vi "Digital Write.vi"(8 "Error In":errorcluster, 9 "Values":bool[](array[boolean]), 10 "Channels":u8[](array[numeric]), 11 "LINX Device Config":T1) -> (0 "Error Out":errorcluster, 3 "LINX Device Config":T1)   [LabVIEW 2013, in "LVH-LINX.lvlib" / "Device.lvlib"]
doc: "Set the value of one or more digital output pin."
uses:
  <vilib>/LabVIEW Hacker/LINX/Private/Device/Device.lvlib
  <vilib>/LabVIEW Hacker/LINX/Private/Device/Type Defs/LINX Device Config.ctl
  <vilib>/LabVIEW Hacker/LINX/Private/Type Defs/Interface.ctl
  <vilib>/LabVIEW Hacker/LINX/Private/Device/Type Defs/TCP Config.ctl
  <vilib>/LabVIEW Hacker/LINX/Private/Type Defs/Device Family.ctl
  <vilib>/LabVIEW Hacker/LINX/Private/Type Defs/Error Type.ctl
  <vilib>/LabVIEW Hacker/LINX/LVH-LINX.lvlib
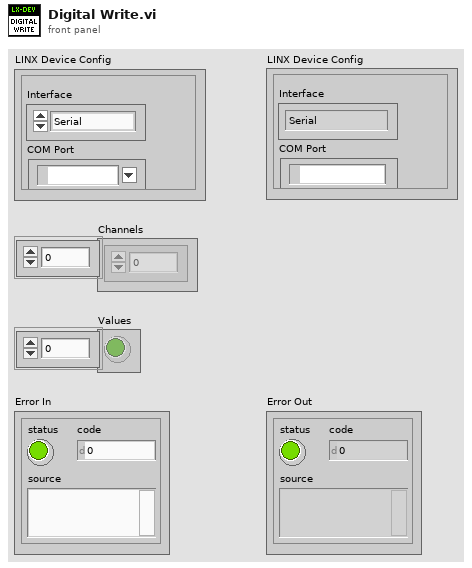
[diagram p1: front panel]
types:
  T1 = typedef "LVH-LINX.lvlib/Device.lvlib/LINX Device Config.ctl" = cluster{"Interface":T2, "COM Port":refnum<visa-resource-name>, "TCP Configuration":T3, "Device Family":T4, "Device ID":u8, "Device Name":string, "TCP Ref":refnum<k5>}
  T2 = typedef "LVH-LINX.lvlib/Interface.ctl" = enum16{"Serial", "TCP"}
  T3 = typedef "LVH-LINX.lvlib/Device.lvlib/TCP Config.ctl" = cluster{"IP Address":string, "Port":u16}
  T4 = typedef "LVH-LINX.lvlib/Device Family.ctl" = enum8{"National Instruments", "Digilent", "Arduino"}
  T5 = typedef "LVH-LINX.lvlib/Error Type.ctl" = enum16{"Unknown", "Timeout", "Corrupt Return Packet", "Unable To Connect", "Command Not Supported", "Channel DNE", "Invalid COM Config"}
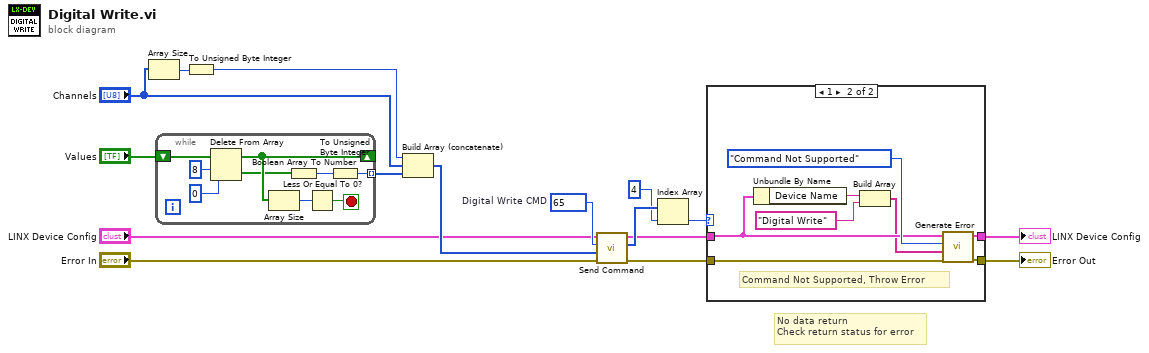
[diagram p0: block diagram]
diagram:
  w15 = u16 65  # Digital Write CMD
  # "No data return\nCheck return status for error"
  n1 = Array Size(array="Channels") -> (size(s)=w14:i32)
  n2 = while {
    shift-right: [w22] -> _
    shift-left: "Values" -> [w25]
    tunnel: [w17] -> w11 mode=indexing
    stop <- w20 stop-if-true
    n3 = Delete From Array(array=w25, length=8 ("index"), index=0 ("length")) -> (deleted portion=w19:bool[], array with subset deleted=w22:bool[])
    n4 = Array Size(array=w22) -> (size(s)=w21:i32)
    n5 = Boolean Array To Number(Boolean array=w19) -> (number=w18:u32)
    n6 = Less Or Equal To 0?(x=w21) -> (x <= 0?=w20:bool)
    n7 = To Unsigned Byte Integer(number=w18) -> (unsigned 8bit integer=w17:u8)
  }
  n8 = To Unsigned Byte Integer(number=w14) -> (unsigned 8bit integer=w13:u8)
  n9 = Build Array (concatenate)(w13, "Channels", w11) -> (w12:u8[])
  n10 = call <vilib>:"Send Command.vi"("Error In"="Error In", "ARGS"=w12, "CMD"=w15, "LINX Device Config"="LINX Device Config") -> ("Error Out"=w5:errorcluster, "Response"=w10:u8[], "LINX Device Config"=w3:T1)  [unwired: 4 in, 1 out]
  n11 = Index Array(array=w10, index=4) -> (element=w8:u8)
  n12 = case shown="1" w8 {
    tunnel: [w27 w33] -> w7
    tunnel: w3 -> [w27 w29]
    tunnel: [w26 w34] -> w6
    tunnel: w5 -> [w26 w35]
    frame 0, Default {
      # "Status OK"
    }
    frame 1 {
      # "Command Not Supported, Throw Error"
      n13 = Unbundle By Name(w29) -> ("Device Name"=w31:string)
      n14 = Build Array(w31, "Digital Write") -> (w28:string[])
      n15 = call <vilib>:"Generate Error.vi"("Error In"=w35, "Arguments"=w28, "Error Type"=Error_Type."Command Not Supported", "LINX Device Config"=w29) -> ("Error Out"=w34:errorcluster, "LINX Device Config"=w33:T1)  [unwired: 6 in]
    }
  }
  "Error Out" <- w6
  "LINX Device Config" <- w7
